vi "Set Sample Rate.vi"(8 "error in (no error)":errorcluster, 10 "Sample Rate":dbl, 11 "Desaccade Manipulator in":refnum<class "Desaccade Manipulator.lvclass">) -> (0 "error out":errorcluster, 3 "Desaccade Manipulator out":refnum<class "Desaccade Manipulator.lvclass">)   [LabVIEW 2016, in "Desaccade Manipulator.lvclass"]
uses:
  Desaccade Manipulator.lvclass
  Desaccade Manipulator.lvclass/Desaccade Manipulator.ctl
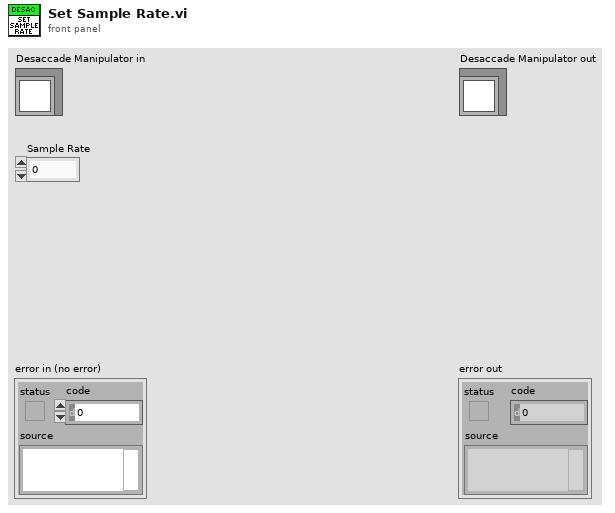
[diagram p1: front panel]
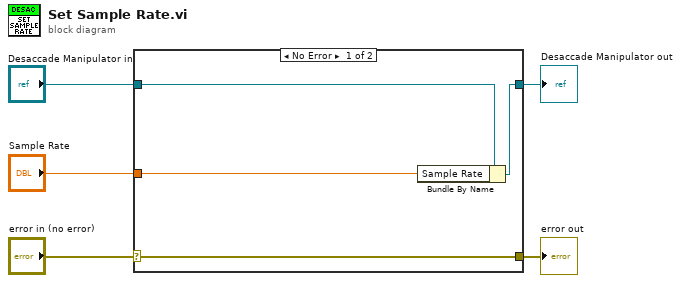
[diagram p0: block diagram]
diagram:
  n1 = case shown="No Error" "error in (no error)" {
    selector: "error in (no error)" -> [w9 w10]
    tunnel: [w9 w10] -> w4
    tunnel: [w7 w11] -> w2
    tunnel: "Desaccade Manipulator in" -> [w8 w11]
    tunnel: "Sample Rate" -> [w6 _]
    frame No Error {
      n2 = Bundle By Name(cluster=w8, "Sample Rate"=w6) -> (w7:refnum<class "Desaccade Manipulator.lvclass">)
    }
    frame Error {
    }
  }
  "error out" <- w4
  "Desaccade Manipulator out" <- w2
